vi "Excel_Set_Page_Numbering.vi"(7 "Include total pages":bool, 8 "error in (no error)":errorcluster, 10 "alignment (right)":u16, 11 "report in":refnum<class "NI_report.lvclass">) -> (0 "error out":errorcluster, 3 "report out":refnum<class "NI_report.lvclass">)   [LabVIEW 2010, in "NI_ReportGenerationToolkit.lvlib"]
uses:
  <vilib>/addons/_office/NI_ReportGenerationToolkit.lvlib
  <vilib>/Utility/NIReport.llb/NI_report.lvclass
  <vilib>/Utility/NIReport.llb/Excel/NI_Excel.lvclass
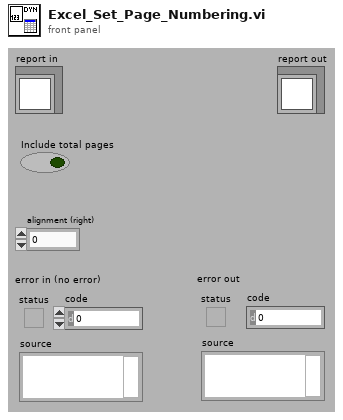
[diagram p1: front panel]
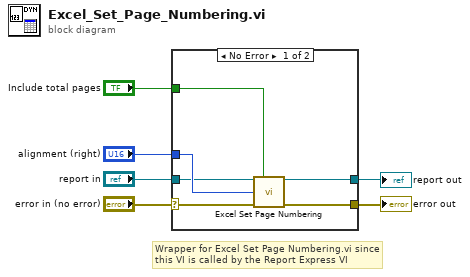
[diagram p0: block diagram]
diagram:
  # "Wrapper for Excel Set Page Numbering.vi since\nthis VI is called by the Report Express VI"
  n1 = case shown="No Error" "error in (no error)" {
    selector: "error in (no error)" -> [w8 w13]
    tunnel: [w12 w13] -> w6
    tunnel: [w11 w14] -> w5
    tunnel: "Include total pages" -> [w10 _]
    tunnel: "alignment (right)" -> [w9 _]
    tunnel: "report in" -> [w7 w14]
    frame No Error {
      n2 = call <vilib>:"Excel Set Page Numbering.vi"("report in"=w7, "include page x of n"=w10, "alignment (right)"=w9, "error in (no error)"=w8) -> ("report out"=w11:refnum<class "NI_report.lvclass">, "error out"=w12:errorcluster)  [unwired: 10 in]
    }
    frame Error {
    }
  }
  "error out" <- w6
  "report out" <- w5
